vi "myRIO_BRig_FPGA_sinwave_getValue.vi"(5 "audioAmp":u16, 6 "sinwave":fxp<+/-,16,2>[](array[numeric]), 7 "audioTrigger":bool, 9 "counter":u32, 10 "k3":fxp<+,18,4>, 11 "k2":u32) -> (0 "output_audioValue":i16, 1 "output_counter":u32)   [LabVIEW 2014]
uses:
  <vilib>/rvi/FXPMathLib/FxpMul/XNode/nifxpmath_Multiplier.xnode
  <vilib>/rvi/FXPMathLib/sim/FxpSim.dll
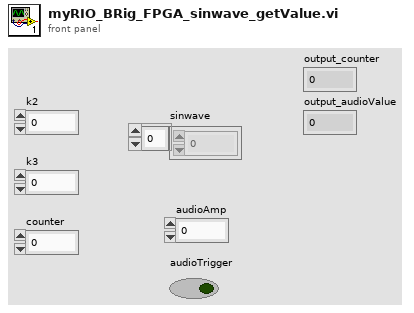
[diagram p1: front panel]
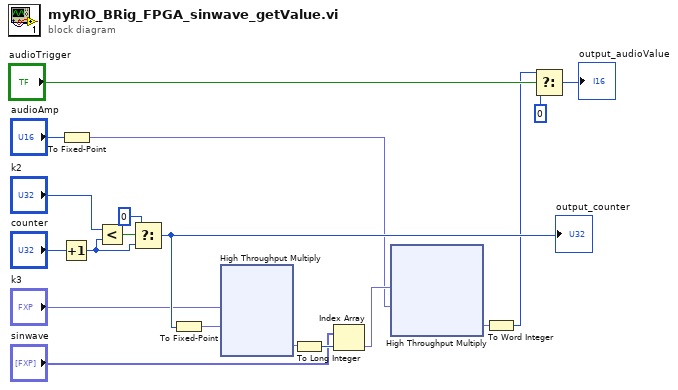
[diagram p0: block diagram]
diagram:
  n1 = Increment(x="counter") -> (x+1=w18:u32)
  n2 = To Fixed-Point(number="audioAmp") -> (fixed-point=w5:fxp<+,15,15>)  [unwired: 1 in]
  n3 = Less?(x="k2", y=w18) -> (x < y?=w19:bool)
  n4 = Select(t=u32 0, s=w19, f=w18) -> (s? t:f=w9:u32)
  "output_counter" <- w9
  n5 = To Fixed-Point(number=w9) -> (fixed-point=w14:fxp<+,32,32>)  [unwired: 1 in]
  n6 = xnode "High Throughput Multiply"("x"="k3", "y"=w14) -> ("x*y"=w13:fxp<+,7,7>)
  n7 = To Long Integer(number=w13) -> (32bit integer=w12:i32)
  n8 = Index Array(array="sinwave", index=w12) -> (element=w10:fxp<+/-,16,2>)
  n9 = xnode ("High Throughput Multiply")("x"=w10, "y"=w5) -> ("x*y"=w11:fxp<+/-,31,17>)
  n10 = To Word Integer(number=w11) -> (16bit integer=w2:i16)
  n11 = Select(t=w2, s="audioTrigger", f=i16 0) -> (s? t:f=→"output_audioValue":i16)
